vi "1_1.vi"() -> ()   [LabVIEW 2025]
panel:
  out "error in (no error)":errorcluster
  out "Answer to Submit":i32
  out "Array":i32[](array[numeric])
  # "Advent Of Code 2021"
  # "Check block diagram for the code"
  # "patrik karandusovsky\npatrik.karandusovsky@gmail.com"
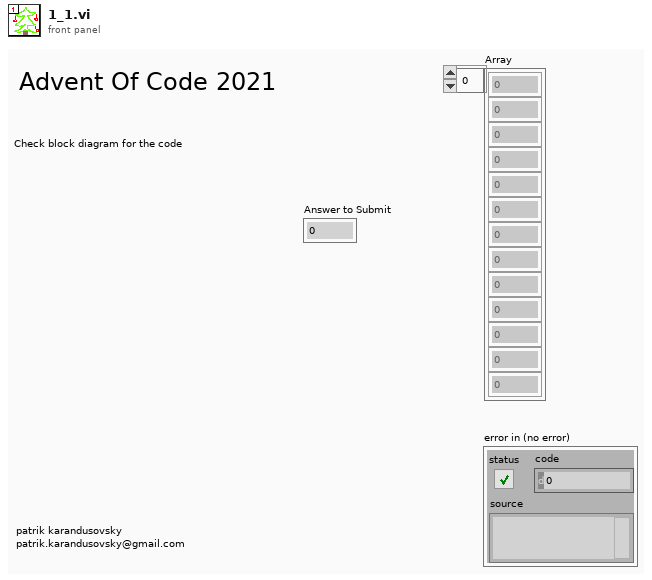
[diagram p1: front panel]
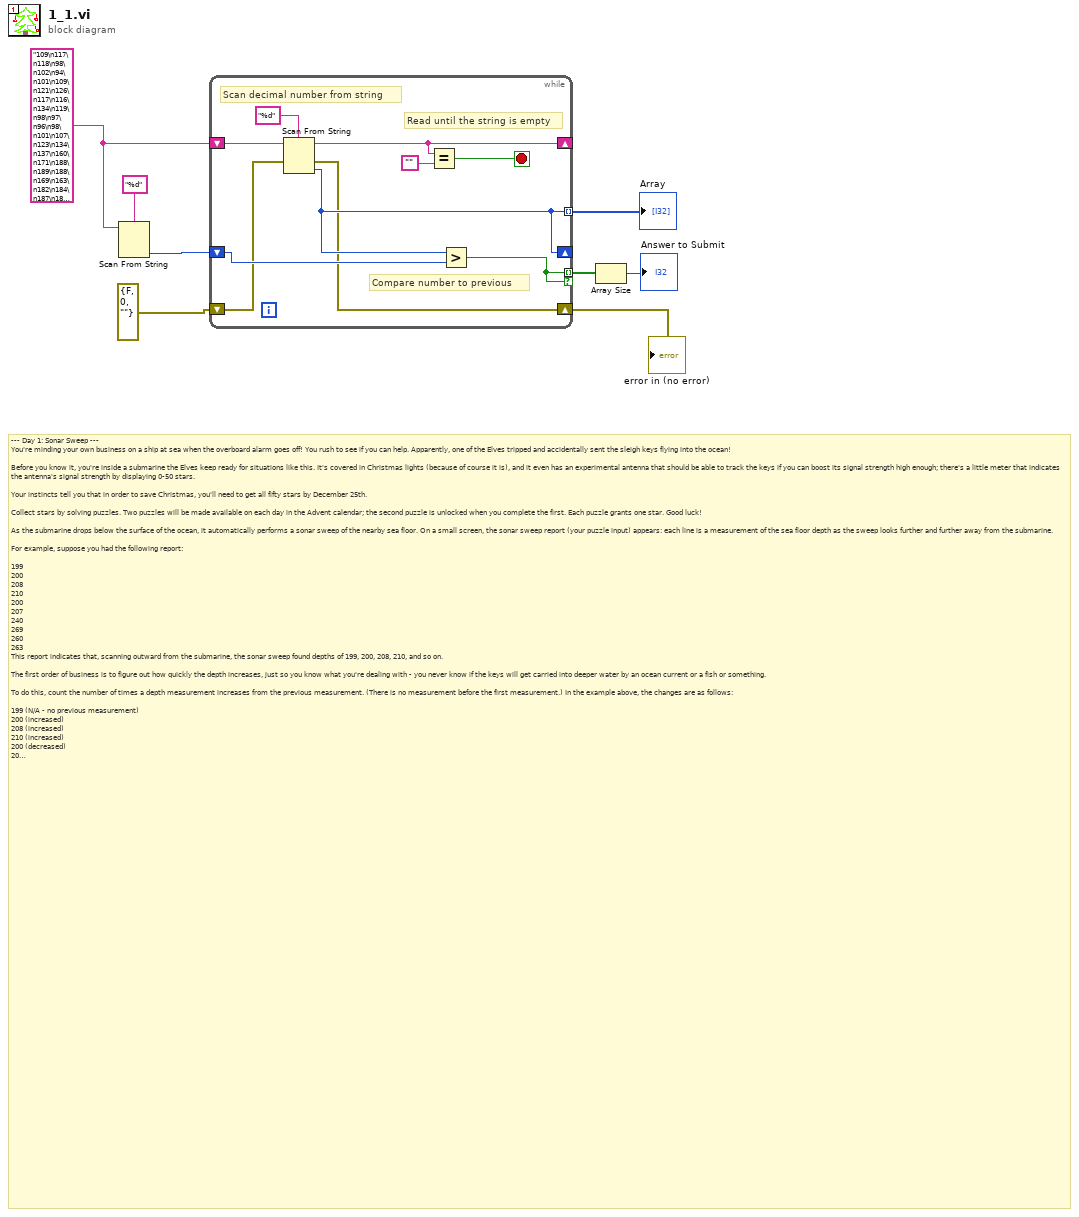
[diagram p0: block diagram]
diagram:
  w7 = "109\n117\n118\n98\n102\n94\n101\n109\n121\n126\n117\n116\n134\n119\n98\n97\n96\n98\n101\n107\n123\n134\n137\n160\n171\n188\n189\n188\n169\n163\n182\n184\n187\n184\n196\n199\n218\n222\n223\n218\n214\n220\n215\n223\n226\n228\n236\n237\n268\n277\n282\n284\n285\n288\n289\n313\n322\n331\n335\n331\n316\n323\n314\n313\n314\n301\n302\n320\n315\n323\n324\n346\n347\n362\n376\n377\n378\n379\n381\n391\n392\n395\n391\n393\n399\n401\n403\n428\n423\n422\n427\n430\n432\n431\n433\n449\n456\n455\n456\n457\n456\n460\n461\n460\n459\n460\n467\n468\n505\n506\n513\n505\n509\n510\n511\n521\n522\n523\n525\n521\n514\n517\n510\n507\n534\n543\n554\n552\n578\n587\n593\n598\n591\n592\n579\n580\n576\n594\n593\n594\n598\n610\n611\n609\n607\n606\n609\n616\n617\n605\n604\n61..." ("Input from adventofcode.com")
  # "--- Day 1: Sonar Sweep ---\nYou're minding your own business on a ship at sea when the overboard alarm goes off! You rush to see if you can help. Apparently, one of the Elves tripped and accidentally sent the sleigh keys flying into the ocean!\n\nBefore you know it, you're inside a submarine the Elves keep ready for situations like this. It's covered in Christmas lights (because of course it is), and it even has an experimental antenna that should be able to track the keys if you can boost its signal strength high enough; there's a little meter that indicates the antenna's signal strength by displaying 0-50 stars.\n\nYour instincts tell you that in order to save Christmas, you'll need to get all fifty stars by December 25th.\n\nCollect stars by solving puzzles. Two puzzles will be made available on each day in the Advent calendar; the second puzzle is unlocked when you complete the first. Each puzzle grants one star. Good luck!\n\nAs the submarine drops below the surface of the ocean, it automatically performs a sonar sweep of the nearby sea floor. On a small screen, the sonar sweep report (your puzzle input) appears: each line is a measurement of the sea floor depth as the sweep looks further and further away from the submarine.\n\nFor example, suppose you had the following report:\n\n199\n200\n208\n210\n200\n207\n240\n269\n260\n263\nThis report indicates that, scanning outward from the submarine, the sonar sweep found depths of 199, 200, 208, 210, and so on.\n\nThe first order of business is to figure out how quickly the depth increases, just so you know what you're dealing with - you never know if the keys will get carried into deeper water by an ocean current or a fish or something.\n\nTo do this, count the number of times a depth measurement increases from the previous measurement. (There is no measurement before the first measurement.) In the example above, the changes are as follows:\n\n199 (N/A - no previous measurement)\n200 (increased)\n208 (increased)\n210 (increased)\n200 (decreased)\n207 (increased)\n240 (increased)\n269 (increased)\n260 (decreased)\n263 (increased)\nIn this example, there are 7 measurements that are larger than the previous measurement.\n\nHow many measurements are larger than the previous measurement?\n\nYour puzzle answer was 1448."
  n1 = Scan From String(format string="%d", input string=w7) -> (output 1=w5:i32)  [unwired: 3 in, 3 out]
  n2 = while {
    shift-right: [w16] -> _
    shift-left: w7 -> [w18]
    tunnel: [w12] -> w8 mode=indexing
    shift-right: [w12] -> _
    shift-left: w5 -> [w13]
    tunnel: [w11] -> w4 mode=indexing if=w11
    shift-right: [w9] -> w1
    shift-left: errorcluster {"status"=FALSE, "code"=0, "source"=""} ("error in (no error)") -> [w10]
    stop <- w14 stop-if-true
    # "Compare number to previous"
    # "Scan decimal number from string"
    # "Read until the string is empty"
    n3 = Scan From String(format string="%d", input string=w18, error in=w10) -> (remaining string=w16:string, error out=w9:errorcluster, output 1=w12:i32)  [unwired: 2 in, 1 out]
    n4 = Equal?(x=w16, y="") -> (x = y?=w14:bool)
    n5 = Greater?(x=w12, y=w13) -> (0:w11:bool)
  }
  "Array" <- w8
  "error in (no error)" <- w1
  n6 = Array Size(array=w4) -> (size(s)=→"Answer to Submit":i32)
